vi "Dummy functional data generator.vi"() -> ()   [LabVIEW 2017]
uses:
  User Interface/Visualisation/Functional Imaging Viewer/SubVIs/Experiment header interface/Typedefs/Header file interface module functions enum.ctl
  Typedefs/Imaging Protocols enum.ctl
  Typedefs/Logging queue element.ctl
  Typedefs/Frame Size.ctl
  Typedefs/Acquired points count.ctl
panel:
  in  "Array":T1[](array[typedef]) {"Ref Dwell time (us)" format="%#.6g"; "Frame Size" items=["100X100"=100, "128X128"=128, "200X200"=200, "256X256"=256, "512X512"=512, "1024x1024"=1024, "2048x2048"=2048]; "Dwell time (us)" format="%#.6g"}
  out "error out":errorcluster
  in  "File path of existing dataset":path=path "C:/Functional Imaging Code/Data_Dummy generated -1POI 1Mscn"
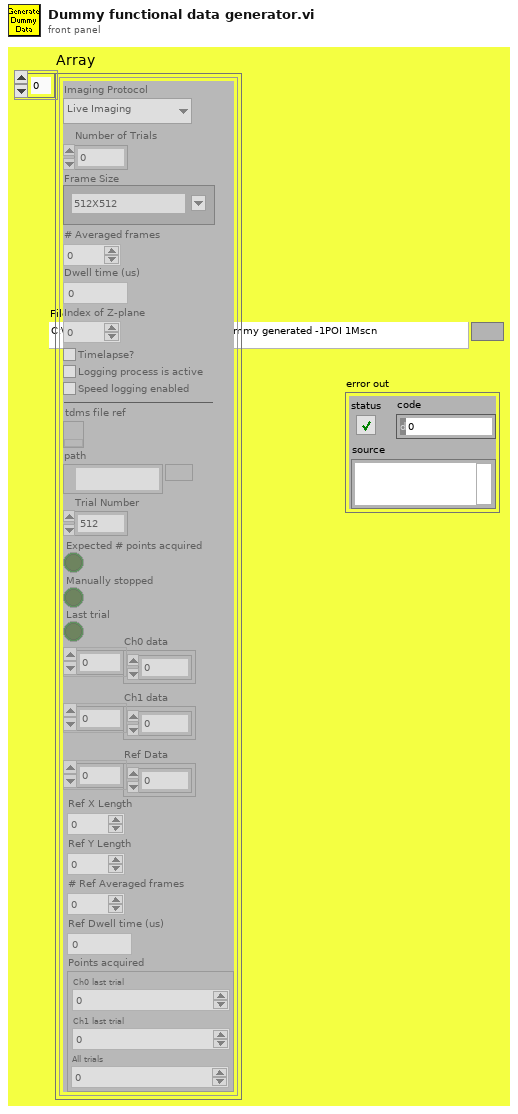
[diagram p1: front panel]
types:
  T1 = typedef "Logging queue element.ctl" = cluster{"Imaging Protocol":T2, "Number of Trials":u16, "Frame Size":T3, "# Averaged frames":u16, "Dwell time (us)":dbl, "Index of Z-plane":i32, "Timelapse?":bool, "Logging process is active":bool, "Speed logging enabled":bool, "tdms file ref":refnum<k34>, "path":path, "Trial Number":i32, "Expected # points acquired":bool, "Manually stopped":bool, "Ch0 data":u32[], "Ch1 data":u32[], "Ref Data":u32[], "Last trial":bool, "Ref Dwell time (us)":dbl, "# Ref Averaged frames":u16, "Ref X Length":u16, "Ref Y Length":u16, "Points acquired":T4}
  T2 = typedef "Imaging Protocols enum.ctl" = enum16{"AOL Z-Stack", "Motor Z Stack", "Functional Acquisition", "Single Plane Acquisition", "Volume Acquisition", "Live Imaging", "Live Plane Imaging", "Live Volume Imaging"}
  T3 = typedef "Frame Size.ctl" = u16
  T4 = typedef "Acquired points count.ctl" = cluster{"Ch0 last trial":u64, "Ch1 last trial":u64, "All trials":u64}
  T5 = typedef "Header file interface module functions enum.ctl" = enum16{"Load experiment header file", "Save experiment header file", "Clear stored values", "Read stored values", "Update specific value in memory", "Update all values in memory"}
  T6 = typedef "Header parameters cluster-ALL.ctl" = cluster{"Imaging Protocol":T2, "Number of POI":u16, "Number of Miniscans":u16, "Number of Trials":u16, "Number of Cycles ":u64, "# Averaged Frames":u16, "Laser power (%)":u8, "Pockels":dbl, "Acquisition Length (sec)":dbl, "Fill time (us)":dbl, "POI Dwell time (us)":dbl, "Miniscan Dwell time per pixel (us)":dbl, "PMT 1":dbl, "PMT 2":dbl, "Back Apperture":dbl, "Zoom":dbl, "Frame Size":T3, "Center Frequency":dbl, "Field of View":dbl, "DwellTime (us)":dbl, "Wavelength (nm)":dbl, "AOL Z":dbl, "AOL Mode":T7, "GridXY":dbl, "GridZ":dbl, "TriggerDelay (sec)":dbl, "Number of Pixels in Miniscan":u16, "Experiment folder path":path, "X centre":dbl, "Y centre":dbl, "Angle (degrees)":dbl, "Plane Mode":T8, "Software version":dbl, "Objective":T9, "MotorZ Calibration":u32, "Pockels Calibration":u32, "Threshold":u16[], "Video length (sec)":dbl, "Frame rate (fps)":u8, "Rectangle ROI length (pixels)":u16, "Rectangle ROI height (pixels)":u16}
  T7 = typedef "AOL modes.ctl" = enum16{"Raster", "Structural", "Pointing", "Mini Scan", "Alignment"}
  T8 = typedef "Plane Mode.ctl" = u16
  T9 = typedef "Objective selector control enum.ctl" = string
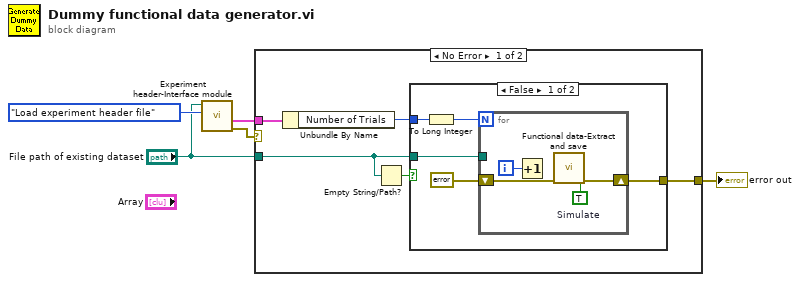
[diagram p0: block diagram]
diagram:
  n1 = call "Experiment header-Interface module.vi"("Function"=Header_file_interface_module_functions_enum."Load experiment header file", "Experiment data folder path"="File path of existing dataset") -> ("error out"=w1:errorcluster, "All header parameters out"=w2:T6)  [unwired: 8 in]
  n2 = case shown="No Error" w1 {
    tunnel: [w10 _] -> w5
    tunnel: "File path of existing dataset" -> [w7 _]
    tunnel: w2 -> [w6 _]
    frame No Error {
      n3 = Unbundle By Name(w6) -> ("Number of Trials"=w8:u16)
      n4 = Empty String/Path?(string/path=w7) -> (empty?=w9:bool)
      n5 = case shown="False" w9 {
        tunnel: w7 -> [w15 _]
        tunnel: w8 -> [w13 _]
        tunnel: [w12 _] -> w10
        frame False {
          n6 = To Long Integer(number=w13) -> (32bit integer=w11:i32)
          n7 = for {
            N: w11 -> [_]
            tunnel: w15 -> [_]
            shift-right: [w19] -> w12
            shift-left: errorcluster {"status"=FALSE, "code"=0, "source"=""} ("error out") -> [w18]
            i -> [w17]
            w16 = TRUE  # Simulate
            n8 = Increment(x=w17) -> ()  [unwired: 1 out]
            n9 = call "Functional data-Extract and save.vi"("Simulate"=w16, "error in (no error)"=w18) -> ("error out"=w19:errorcluster)  [unwired: 8 in, 1 out]
          }
        }
        frame True {
        }
      }
    }
    frame Error {
    }
  }
  "error out" <- w5
